vi "_setDecorationRef.vi"(7 "parentURL":string, 8 "error in (no error)":errorcluster, 9 "Name":string, 10 "Refnum":refnum<vi>, 11 "TagDB in":refnum<k1>) -> (0 "error out":errorcluster, 2 "URL":string, 3 "TagDB out":refnum<k1>)   [LabVIEW 2017, in "TagDB RefManager.lvlib"]
uses:
  TagDB RefManager.lvlib
  49cb8d7b-d4e1-40e6-a881-9df98b6c0263.vi
  <userlib>/_NEVSTOP/TagDB/_Support/DataAccess/data-Write.vi
  <userlib>/_NEVSTOP/TagDB/_Support/Error/_[error50000]Invalid DB REF.vi
  <userlib>/_NEVSTOP/TagDB/_Support/DataAccess/TagDB Ref to DVR.vi
  <userlib>/_NEVSTOP/TagDB/_Support/DataAccess/_NameCacher.vi
  <userlib>/_NEVSTOP/TagDB/_Support/DataAccess/_datatypeChecker.vi
  <userlib>/_NEVSTOP/TagDB/_Support/Error/_Build Error Cluster.vi
  <vilib>/Utility/Data Type/Get Type Information.vi
  <userlib>/_NEVSTOP/TagDB/TagDB.lvlib
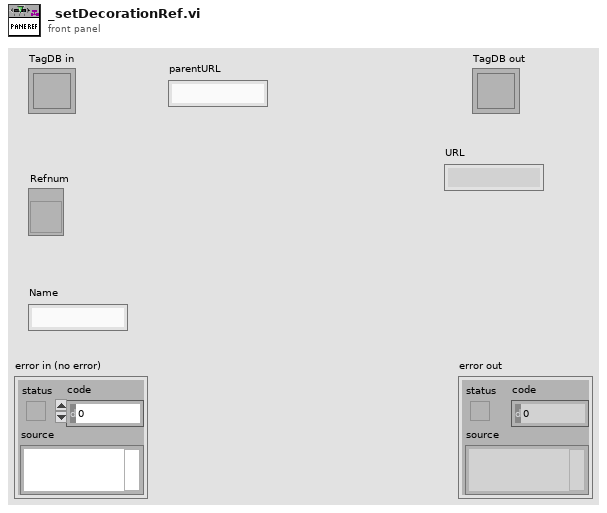
[diagram p1: front panel]
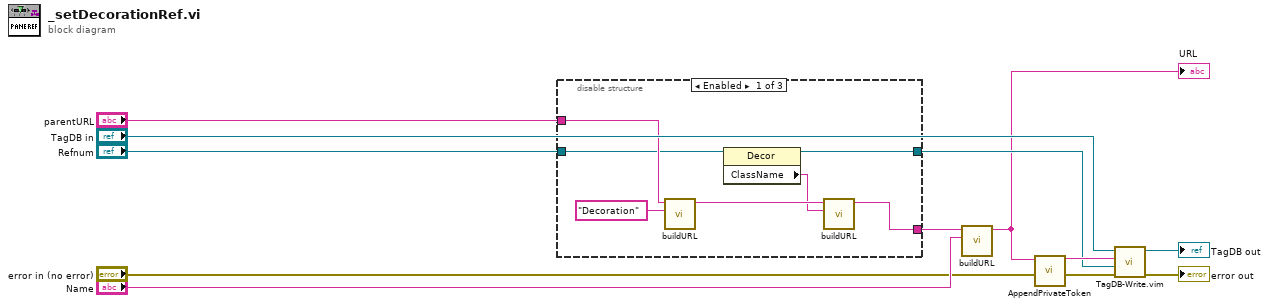
[diagram p0: block diagram]
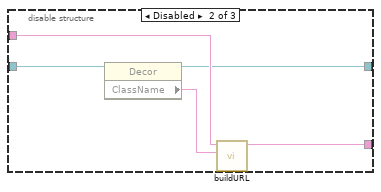
[diagram p2: hidden frame]
diagram:
  n1 = disable-structure shown="Enabled" {
    disable-tunnel: [w13 w23 w24] -> w10
    disable-tunnel: "parentURL" -> [w18 w22 w24]
    disable-tunnel: "Refnum" -> [w16 w21 w25]
    disable-tunnel: [w15 w20 w25] -> w2
    frame Enabled {
      n2 = call <userlib>:"buildURL.vi"("DataName"="Decoration", "parentURL"=w18) -> ("DataURL"=w14:string)  [unwired: 9 in]
      n3 = property class="Decor"(reference=w16) -> (reference out=w15:refnum<vi>, "ClassName"=w12:string)  [unwired: 1 in, 1 out]
      n4 = call <userlib>:"buildURL.vi"("DataName"=w12, "parentURL"=w14) -> ("DataURL"=w13:string)  [unwired: 9 in]
    }
    frame Disabled {
      n5 = property class="Decor"(reference=w21) -> (reference out=w20:refnum<vi>, "ClassName"=w19:string)  [unwired: 1 in, 1 out]
      n6 = call <userlib>:"buildURL.vi"("DataName"=w19, "parentURL"=w22) -> ("DataURL"=w23:string)  [unwired: 9 in]
    }
    frame Disabled {
    }
  }
  n7 = call <userlib>:"buildURL.vi"("DataName"="Name", "parentURL"=w10) -> ("DataURL"=w1:string)  [unwired: 9 in]
  "URL" <- w1
  n8 = call <userlib>:"AppendPrivateToken.vi"("DataURL"=w1) -> ("String"=w3:string)  [unwired: 10 in]
  n9 = call "TagDB-Write.vim"("error in (no error)"="error in (no error)", "Value"=w2, "tag"=w3, "TagDB"="TagDB in") -> ("error out"=→"error out":errorcluster, "TagDB(dup)"=→"TagDB out":refnum<k1>)  [unwired: 5 in, 1 out]
